vi "e.gate HighSpeedPort Read Buffer.vi"(0 "e.gate Configuration In":T1, 5 "Backtime":dbl, 7 "Iteration":i32=1000, 9 "force Backtime":bool, 11 "error in (no error)":errorcluster, 12 "No Erasing":bool, 13 "DecodeTimeFormat":string) -> (4 "e.gate Configuration Out":T1, 6 "Value":dbl[][](array[numeric]), 15 "error out":errorcluster)   [LabVIEW 2016]
doc: "<B>AMC - Analytik & Messtechnik GmbH Chemnitz</B>\n\nLabVIEW Drivers for e.gate / e.pac series from Gantner Instruments\n\nThis VI reads a value specified by <B>Channel</B> from a device specified by <B>connection ID In</B>."
uses:
  e.gate Configuration.ctl
  e.gate Channel Data.ctl
  e.gate Data Type.ctl
  e.gate Protocol Type.ctl
  e.gate Module  Data.ctl
  e.gateHSP_DLLhandle.ctl
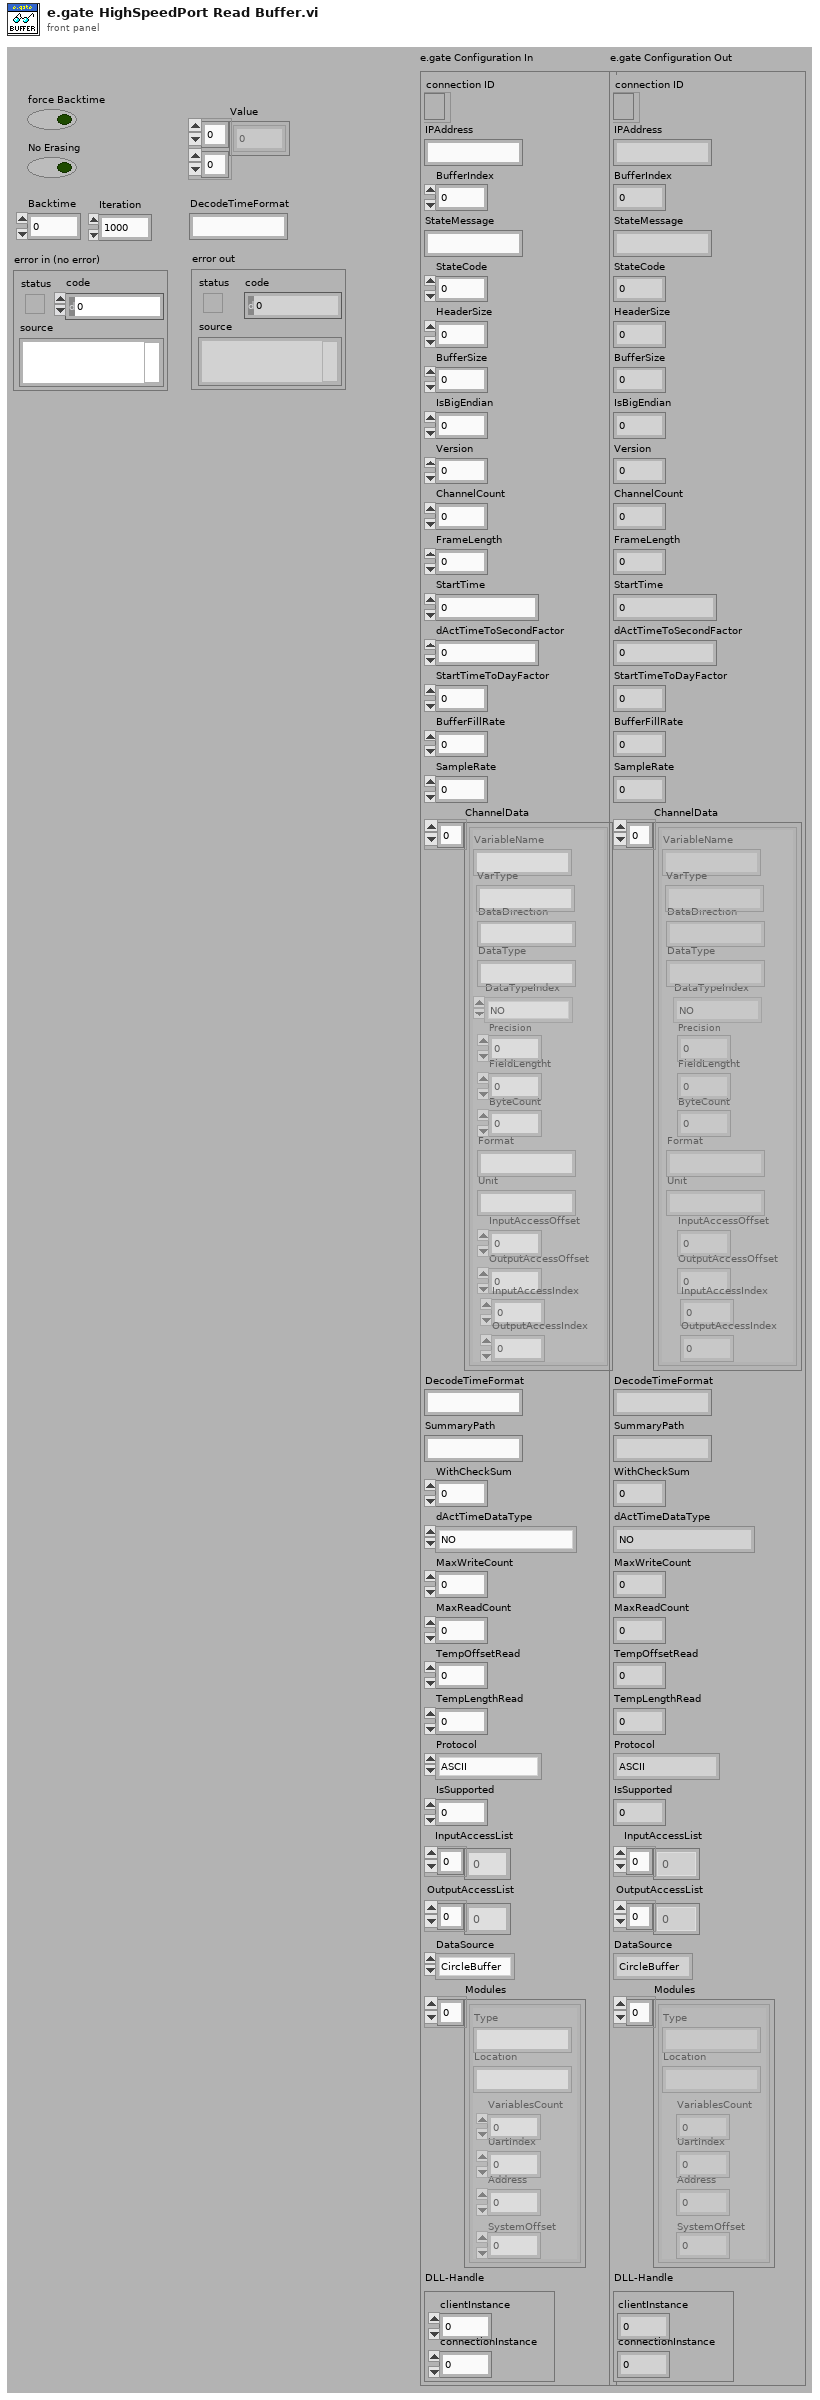
[diagram p1: front panel]
types:
  T1 = typedef "e.gate Configuration.ctl" = cluster{"connection ID":refnum<k5>, "IPAddress":string, "BufferIndex":i32, "StateMessage":string, "StateCode":i8, "HeaderSize":i32, "BufferSize":i32, "IsBigEndian":i32, "Version":i32, "ChannelCount":i32, "FrameLength":i32, "StartTime":dbl, "dActTimeToSecondFactor":dbl, "StartTimeToDayFactor":dbl, "BufferFillRate":dbl, "SampleRate":dbl, "ChannelData":T2[], "DecodeTimeFormat":string, "SummaryPath":string, "WithCheckSum":i32, "dActTimeDataType":T3, "MaxWriteCount":i32, "MaxReadCount":i32, "TempOffsetRead":i32, "TempLengthRead":i32, "Protocol":T4, "IsSupported":i32, "InputAccessList":i32[], "OutputAccessList":i32[], "DataSource":enum16{"CircleBuffer", "test.con Logger", "test.con Archive"}, "Modules":T5[], "DLL-Handle":T6}
  T2 = typedef "e.gate Channel Data.ctl" = cluster{"VariableName":string, "DataDirection":string, "DataType":string, "DataTypeIndex":T3, "Precision":i16, "FieldLengtht":i16, "ByteCount":i32, "Format":string, "Unit":string, "InputAccessOffset":i32, "OutputAccessOffset":i16, "InputAccessIndex":i16, "OutputAccessIndex":i16, "VarType":string}
  T3 = typedef "e.gate Data Type.ctl" = enum16{"NO", "BOOL", "SINT8", "USINT8", "SINT16", "USINT16", "SINT32", "USINT32", "FLOAT", "SET8", "SET16", "SET32", "DOUBLE", "SINT64", "USINT64", "SET64"}
  T4 = typedef "e.gate Protocol Type.ctl" = enum16{"ASCII", "HighspeedPort Online", "HighspeedPort Buffer", "eGateHighspeedPortDLL "}
  T5 = typedef "e.gate Module  Data.ctl" = cluster{"Type":string, "Location":string, "VariablesCount":i16, "UartIndex":i16, "Address":i16, "SystemOffset":i16}
  T6 = typedef "e.gateHSP_DLLhandle.ctl" = cluster{"clientInstance":i32, "connectionInstance":i32}
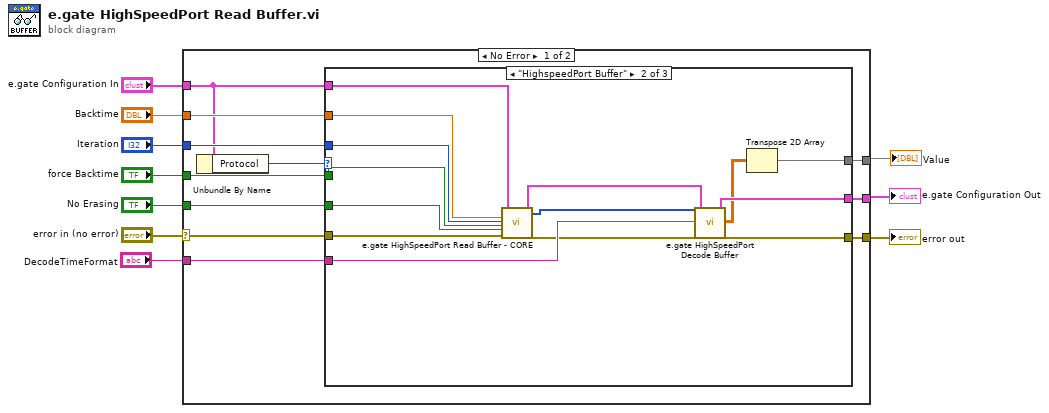
[diagram p0: block diagram]
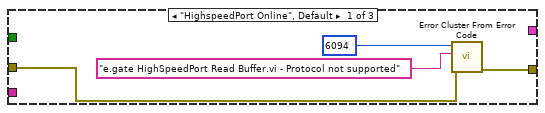
[diagram p2: hidden frame]
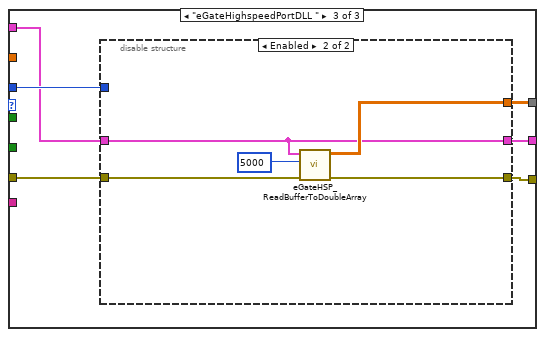
[diagram p3: hidden frame]
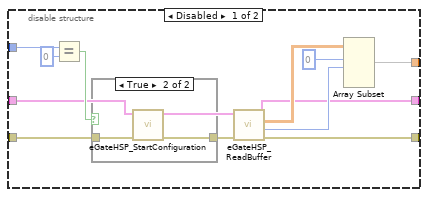
[diagram p4: hidden frame]
diagram:
  n1 = case shown="No Error" "error in (no error)" {
    selector: "error in (no error)" -> [w14 w67]
    tunnel: "e.gate Configuration In" -> [w12 w66]
    tunnel: [w21 w66] -> w8
    tunnel: [w13 w67] -> w7
    tunnel: [w15 _] -> w6
    tunnel: "Backtime" -> [w20 _]
    tunnel: "Iteration" -> [w19 _]
    tunnel: "force Backtime" -> [w18 _]
    tunnel: "No Erasing" -> [w17 _]
    tunnel: "DecodeTimeFormat" -> [w16 _]
    frame No Error {
      n2 = Unbundle By Name(w12) -> ("Protocol"=w11:T4)
      n3 = case shown="\"HighspeedPort Buffer\"" w11 {
        tunnel: [_ w39 w41] -> w21
        tunnel: w12 -> [_ w38 w43]
        tunnel: w20 -> [_ w35 _]
        tunnel: w19 -> [_ w34 w45]
        tunnel: w18 -> [_ w33 _]
        tunnel: w17 -> [_ w32 _]
        tunnel: w16 -> [_ w31 _]
        tunnel: [_ w29 w42] -> w15
        tunnel: w14 -> [w24 w28 w44]
        tunnel: [w23 w26 w40] -> w13
        frame "HighspeedPort Online", Default {
          n4 = call <vilib>:"Error Cluster From Error Code.vi"("error in (no error)"=w24, "error message (\"\")"="e.gate HighSpeedPort Read Buffer.vi - Protocol not supported" ("error message (\"\")"), "error code (0)"=i16 6094 ("y")) -> ("error out"=w23:errorcluster)  [unwired: 1 in, 5 out]
        }
        frame "HighspeedPort Buffer" {
          n5 = call "e.gate HighSpeedPort Read Buffer - CORE.vi"("Backtime"=w35, "Iteration"=w34, "force Backtime"=w33, "No Erasing"=w32, "error in (no error)"=w28, "Configuration in"=w38) -> ("Configuration out"=w37:T1, "data array (binary)"=w36:u8[], "error out"=w27:errorcluster)  [unwired: 19 out]
          n6 = call "e.gate HighSpeedPort Decode Buffer.vi"("Data in (binary)"=w36, "DecodeTimeFormat"=w31, "error in"=w27, "Configuration  in"=w37) -> ("Configuration out"=w39:T1, "data array (double)"=w30:dbl[][], "error out"=w26:errorcluster)  [unwired: 21 out]
          n7 = Transpose 2D Array(2D array=w30) -> (transposed array=w29:dbl[][])
        }
        frame "eGateHighspeedPortDLL " {
          n8 = disable-structure shown="Enabled" {
            disable-tunnel: w45 -> [w57 _]
            disable-tunnel: w44 -> [w54 w61]
            disable-tunnel: w43 -> [w52 w62]
            disable-tunnel: [w48 w63] -> w42
            disable-tunnel: [w47 w62] -> w41
            disable-tunnel: [w46 w64] -> w40
            frame Disabled {
              n9 = Equal?(x=w57, y=0) -> (x = y?=w55:bool)
              n10 = case shown="True" w55 {
                tunnel: w54 -> [w58 w60]
                tunnel: [w58 w59] -> w53
                frame False {
                }
                frame True {
                  n11 = call "eGateHSP_StartConfiguration.vi"("Fehler (Eingang, kein Fehler)"=w60) -> ("Fehler (Ausgang)"=w59:errorcluster)  [unwired: 10 in]
                }
              }
              n12 = call "eGateHSP_ReadBuffer.vi"("Fehler (Eingang, kein Fehler)"=w53, "e.gate Configuration"=w52) -> ("Fehler (Ausgang)"=w46:errorcluster, "number of Frames"=w50:i32, "Array"=w51:dbl[][], "e.gate Configuration 2"=w47:T1)  [unwired: 4 in]
              n13 = Array Subset(array=w51, index (row)=0 ("Index"), length (row)=w50) -> (w48:dbl[][])  [unwired: 2 in]
            }
            frame Enabled {
              n14 = call "eGateHSP_ReadBufferToDoubleArray.vi"("Fehler (Eingang, kein Fehler)"=w61, "NumberOfFrames"=5000, "e.gate Configuration"=w62) -> ("Fehler (Ausgang)"=w64:errorcluster, "Array (Ausgang)"=w63:dbl[][])  [unwired: 7 in]
            }
          }
        }
      }
    }
    frame Error {
    }
  }
  "error out" <- w7
  "e.gate Configuration Out" <- w8
  "Value" <- w6
